vi "CMD_GETPOS.vi"(6 "Gantry in":refnum<class "Gantry.lvclass">, 8 "error in (no error)":errorcluster, 10 "Arguments":string[](array[string]), 11 "gScript Interpreter in":refnum<class "gScript Interpreter.lvclass">) -> (0 "error out":errorcluster, 3 "gScript Interpreter out":refnum<class "gScript Interpreter.lvclass">, 4 "Gantry out":refnum<class "Gantry.lvclass">)   [LabVIEW 2024, in "gScript Interpreter.lvclass"]
uses:
  gScript Interpreter.lvclass
  Shared Components/Gantry Class/Gantry.lvclass
  Type Definitions/Memory Cell.ctl
  Type Definitions/Memory Cell Type Enum.ctl
  Shared Components/Vec3d Class/Vec3d.lvclass
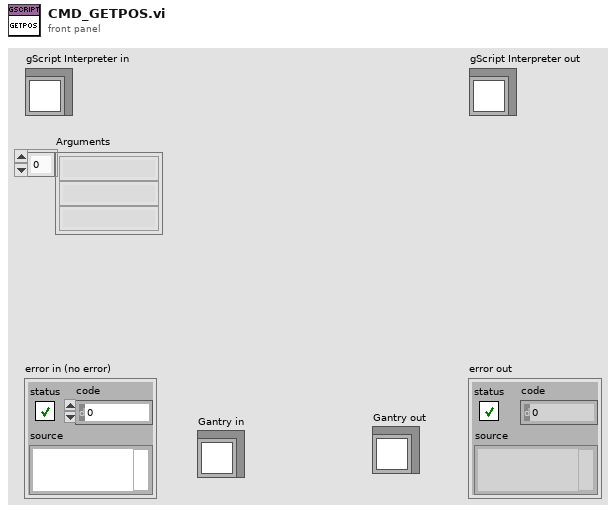
[diagram p1: front panel]
types:
  T1 = typedef "Memory Cell Type Enum.ctl" = enum16{"integer", "float", "vector", "rotation"}
  T2 = typedef "Memory Cell.ctl" = cluster{"type":T1, "x":dbl, "y":dbl, "z":dbl, "w":dbl}
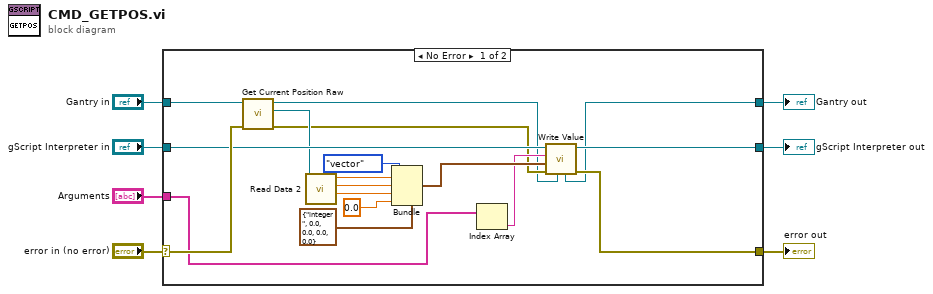
[diagram p0: block diagram]
diagram:
  n1 = case shown="No Error" "error in (no error)" {
    selector: "error in (no error)" -> [w24 w28]
    tunnel: [w10 w28] -> w6
    tunnel: [w22 w27] -> w4
    tunnel: "gScript Interpreter in" -> [w23 w27]
    tunnel: "Arguments" -> [w13 _]
    tunnel: "Gantry in" -> [w25 w26]
    tunnel: [w8 w26] -> w1
    frame No Error {
      n2 = call-dynamic "Get Current Position Raw.vi"("error in"=w24, "Gantry in"=w25) -> ("error out"=w11:errorcluster, "Vec3d Class out"=w20:refnum<class "Vec3d.lvclass">, "Gantry out"=w9:refnum<class "Gantry.lvclass">)  [unwired: 7 in]
      n3 = call-dynamic "Read Data 2.vi"("Vec3d in"=w20) -> ("Z"=w17:dbl, "Y"=w18:dbl, "X"=w19:dbl)  [unwired: 7 in, 1 out]
      n4 = Bundle(cluster=T2 {"type"=enum."integer", "x"=0.0, "y"=0.0, "z"=0.0, "w"=0.0} ("Value"), "type"=Memory_Cell_Type_Enum."vector", "x"=w19, "y"=w18, "z"=w17, "w"=0.0) -> (w14:T2)
      n5 = Index Array(array=w13) -> (element=w12:string)  [unwired: 1 in]
      n6 = call-dynamic "Write Value.vi"("Gantry in"=w9, "error in (no error)"=w11, "Value"=w14, "Address"=w12, "gScript Interpreter in"=w23) -> ("error out"=w10:errorcluster, "gScript Interpreter out"=w22:refnum<class "gScript Interpreter.lvclass">, "Gantry out"=w8:refnum<class "Gantry.lvclass">)  [unwired: 4 in]
    }
    frame Error {
    }
  }
  "error out" <- w6
  "gScript Interpreter out" <- w4
  "Gantry out" <- w1
